vi "Initialise Test Data.vi"(8 "error in (no error)":errorcluster, 11 "Test in":refnum<class "Test.lvclass">) -> (0 "error out":errorcluster, 3 "Test out":refnum<class "Test.lvclass">)   [LabVIEW 2018, in "Test.lvclass"]
doc: "Configures all the fixed test values and preinitialises other values to known data to allow a test to be built"
uses:
  Test.lvclass
  Test.lvclass/Test.ctl
  Test Class String IDs.vi
panel:
  out "<JSON>":string
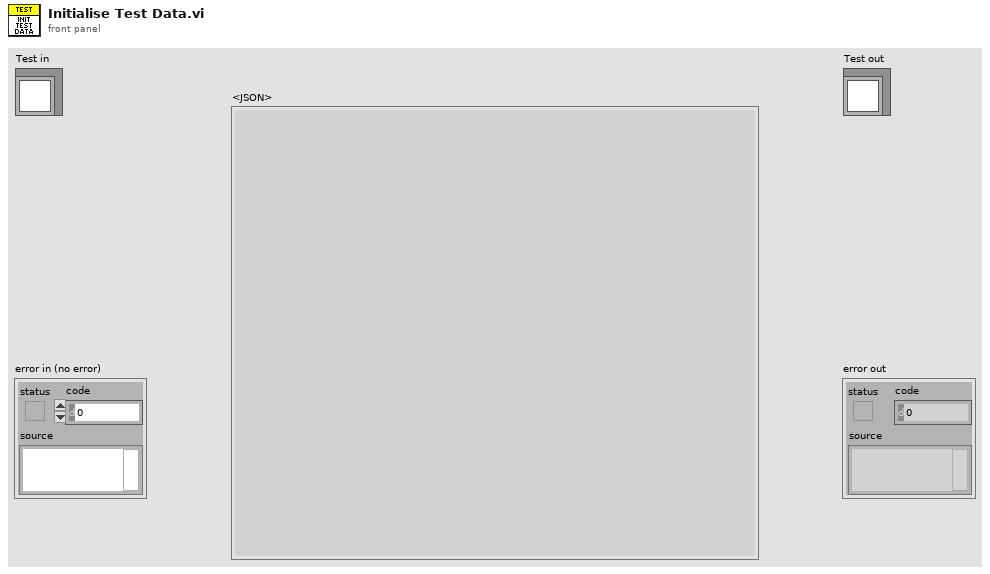
[diagram p1: front panel]
types:
  T1 = enum16{"Display Only", "Log To File", "Pause Execution", "Abort Execution"}
  T2 = cluster{"Comparison Value 1":string, "Comparison Value 2":string, "Invert Result":string, "Assert VI Name":string, "Data Type":string, "Builder User Name":string, "Build Timestamp":string, "Failure Action":string, "Comment":string, "Assert Name":string, "Description":string, "Evaluation String":string}
  T3 = typedef "NI_Data Type.lvlib/Data Type.ctl" = enum8{"Invalid Type", "Void", "I8", "I16", "I32", "I64", "U8", "U16", "U32", "U64", "Single Float", "Double Float", "Extended Float", "Single Complex", "Double Complex", "Extended Complex", "Enum U8", "Enum U16", "Enum U32", "Enum U64", "Single Float With Unit", "Double Float With Unit", "Extended Float With Unit", "Single Complex with Unit", "Double Complex with Unit", "Extended Complex with Unit", "Boolean", "String", "Path", "Picture", "Tag", "Array", "Cluster", "Variant", "LV Variant", "Waveform", "Timestamp", "Digital Waveform", "Digital Data", "ExpressData", "Refnum", "External Data", "VI", "Poly VI", "LabVIEW Class Instance", "Fixed Point"}
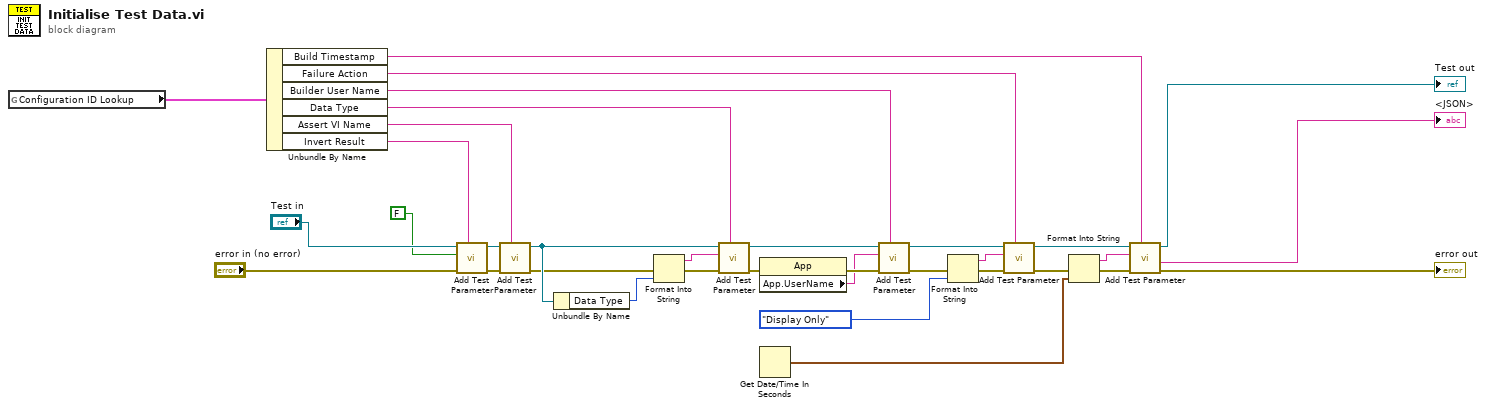
[diagram p0: block diagram]
diagram:
  n1 = global read "Test Class String IDs.vi" "Configuration ID Lookup"() -> (w34:T2)
  n2 = Unbundle By Name(w34) -> ("Build Timestamp"=w16:string, "Failure Action"=w13:string, "Builder User Name"=w25:string, "Data Type"=w26:string, "Assert VI Name"=w27:string, "Invert Result"=w28:string)
  n3 = call-dynamic "Add Test Parameter.vi"("Data Value ID"=w28, "error in (no error)"="error in (no error)", "Data Value"=FALSE, "Test in"="Test in") -> ("error out"=w32:errorcluster, "Test out"=w33:refnum<class "Test.lvclass">)  [unwired: 5 in, 1 out]
  n4 = call-dynamic "Add Test Parameter.vi"("Data Value ID"=w27, "error in (no error)"=w32, "Test in"=w33) -> ("error out"=w4:errorcluster, "Test out"=w21:refnum<class "Test.lvclass">)  [unwired: 6 in, 1 out]
  n5 = Unbundle By Name(w21) -> ("Data Type"=w3:T3)
  n6 = Format Into String(error in=w4, w3) -> (resulting string=w1:string, error out=w2:errorcluster)  [unwired: 2 in]
  n7 = call-dynamic "Add Test Parameter.vi"("Data Value ID"=w26, "error in (no error)"=w2, "Data Value"=w1, "Test in"=w21) -> ("error out"=w24:errorcluster, "Test out"=w31:refnum<class "Test.lvclass">)  [unwired: 5 in, 1 out]
  n8 = property class="App"(error in=w24) -> (error out=w23:errorcluster, "App.UserName"=w22:string)  [unwired: 1 in, 1 out]
  n9 = Get Date/Time In Seconds() -> (seconds since 1Jan1904=w8:timestamp)
  n10 = call-dynamic "Add Test Parameter.vi"("Data Value ID"=w25, "error in (no error)"=w23, "Data Value"=w22, "Test in"=w31) -> ("error out"=w10:errorcluster, "Test out"=w15:refnum<class "Test.lvclass">)  [unwired: 5 in, 1 out]
  n11 = Format Into String(error in=w10, T1."Display Only" ("Default Failure Action")) -> (resulting string=w11:string, error out=w9:errorcluster)  [unwired: 2 in]
  n12 = call-dynamic "Add Test Parameter.vi"("Data Value ID"=w13, "error in (no error)"=w9, "Data Value"=w11, "Test in"=w15) -> ("error out"=w7:errorcluster, "Test out"=w14:refnum<class "Test.lvclass">)  [unwired: 5 in, 1 out]
  n13 = Format Into String(error in=w7, w8) -> (resulting string=w5:string, error out=w6:errorcluster)  [unwired: 2 in]
  n14 = call-dynamic "Add Test Parameter.vi"("Data Value ID"=w16, "error in (no error)"=w6, "Data Value"=w5, "Test in"=w14) -> ("error out"=→"error out":errorcluster, "<JSON>"=→"<JSON>":string, "Test out"=→"Test out":refnum<class "Test.lvclass">)  [unwired: 5 in]
